vi "ThreePts_PlainEqn.vi"(2 "V3":dbl[](array[numeric]), 3 "V2":dbl[](array[numeric]), 4 "V1":dbl[](array[numeric])) -> (0 "D":dbl format="%.2f", 1 "Normal Vector (A B C)":dbl[](array[numeric]))   [LabVIEW 2016, in "ForceField.lvclass"]
uses:
  ForceField.lvclass
  <vilib>/Analysis/baseanly.llb/Real Dot Product.vi
  <vilib>/Analysis/NI_AALPro.lvlib
  <vilib>/Analysis/NI_AALBase.lvlib
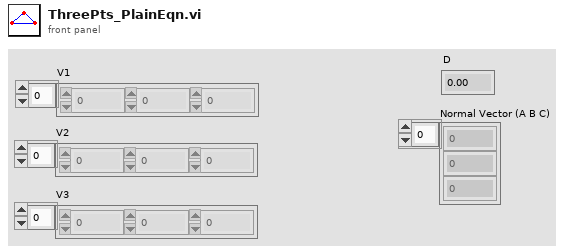
[diagram p1: front panel]
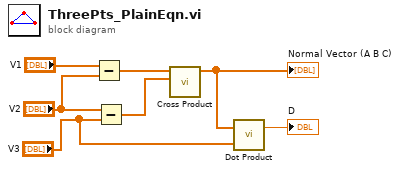
[diagram p0: block diagram]
diagram:
  n1 = Subtract(x="V1", y="V2") -> (x-y=w7:dbl[])
  n2 = Subtract(x="V2", y="V3") -> (x-y=w6:dbl[])
  n3 = call <vilib>:"Cross Product.vi"("B Vector"=w6, "A Vector"=w7) -> ("Cross Product"=w5:dbl[])  [unwired: 8 in, 1 out]
  "Normal Vector (A B C)" <- w5
  n4 = call-poly <vilib>:"Dot Product.vi"("Y Vector"="V3", "X Vector"=w5) -> ("X * Y"=→"D":dbl)  [unwired: 1 out]
